vi "String to Int.vi"(11 "String":string) -> (3 "I32":i32)   [LabVIEW 2024, in "EDS.lvlib"]
doc: "Converts the string representation of a number in a specified base to an equivalent 32-bit signed integer."
uses:
  EDS.lvlib
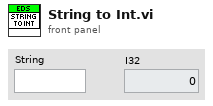
[diagram p1: front panel]
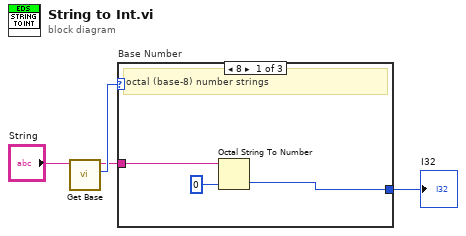
[diagram p0: block diagram]
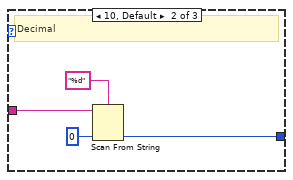
[diagram p2: hidden frame]
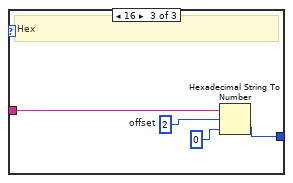
[diagram p3: hidden frame]
diagram:
  n1 = call "Get Base.vi"("Default Value"="String") -> ("Number Base"=w2:u8, "Default Value (dup)"=w1:string)  [unwired: 9 in]
  n2 = case "Base Number" shown="8" w2 {
    tunnel: [w5 w8 w15] -> w4
    tunnel: w1 -> [w7 w11 w12]
    frame 8 {
      # "octal (base-8) number strings"
      n3 = Octal String To Number(2:i16 0 ("offset (0)"), 4:w7) -> (0:w5:i16)  [unwired: 1 in, 1 out]
    }
    frame 10, Default {
      # "Decimal"
      n4 = Scan From String(format string="%d", input string=w11, default 1=0) -> (output 1=w8:i32)  [unwired: 2 in, 3 out]
    }
    frame 16 {
      w13 = 2  # offset
      # "Hex"
      n5 = Hexadecimal String To Number(string=w12, offset=w13, default (0uL)=i16 0 ("offset (0)")) -> (number=w15:i16)  [unwired: 1 out]
    }
  }
  "I32" <- w4
